vi "Globavl float VI.vi"(3 "Set Value?":bool, 9 "New Value":dbl) -> (1 "Current value":dbl, 11 "Boolean":bool)   [LabVIEW 2018]
doc: "Shift register VI"
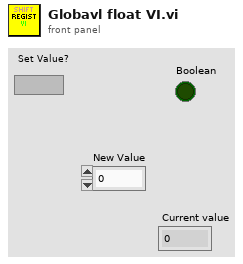
[diagram p1: front panel]
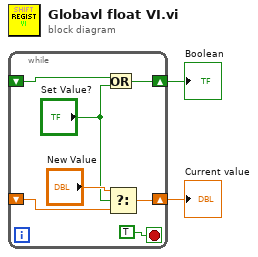
[diagram p0: block diagram]
diagram:
  n1 = while {
    shift-right: [w8] -> w2
    shift-left: _ -> [w7]
    shift-right: [w4] -> w1
    shift-left: _ -> [w3]
    stop <- TRUE stop-if-true
    n2 = Or(x=w3, y="Set Value?") -> (x .or. y?=w4:bool)
    n3 = Select(t="New Value", s="Set Value?", f=w7) -> (s? t:f=w8:dbl)
  }
  "Boolean" <- w1
  "Current value" <- w2
